vi "CHROMA Set Coupling.vi"(8 "Error In":errorcluster, 10 "Chroma Couple":T1, 11 "CHROMA VISA In":refnum<visa-resource-name>) -> (0 "Error Out":errorcluster, 3 "CHROMA VISA Out":refnum<visa-resource-name>)   [LabVIEW 2020]
uses:
  Type Definition/CHROMA Set Coupling.ctl
  Type Definition/CHROMA Build CMD Type.ctl
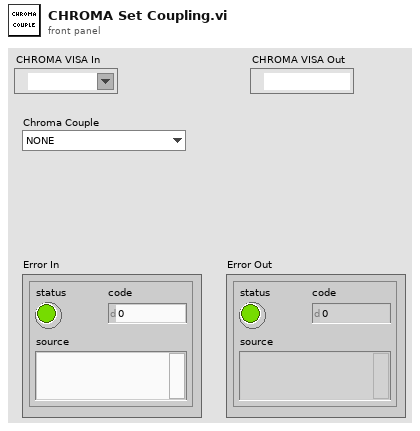
[diagram p1: front panel]
types:
  T1 = typedef "CHROMA Set Coupling.ctl" = enum16{"NONE", "ALL"}
  T2 = typedef "CHROMA Build CMD Type.ctl" = enum16{"Value DBL", "Value I32", "String"}
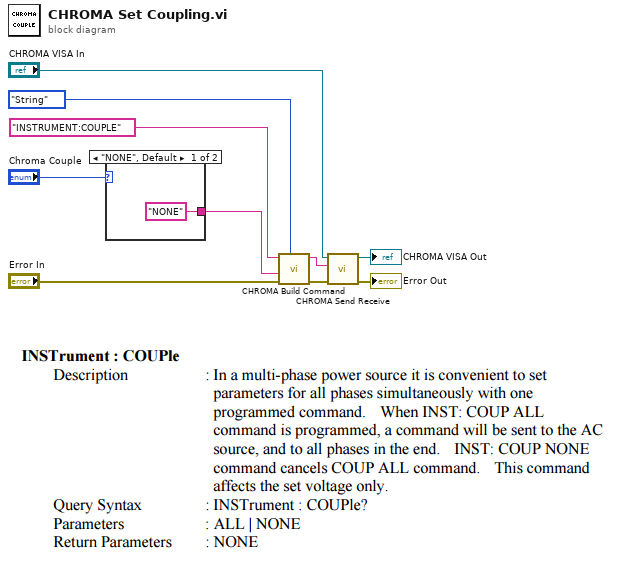
[diagram p0: block diagram]
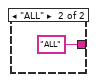
[diagram p2: hidden frame]
diagram:
  n1 = case shown="\"NONE\", Default" "Chroma Couple" {
    tunnel: ["NONE" "ALL"] -> w6
    frame "NONE", Default {
    }
    frame "ALL" {
    }
  }
  n2 = call "CHROMA Build Command.vi"("Build Type"=CHROMA_Build_CMD_Type."String", "Error In"="Error In", "String"=w6, "Partial Command"="INSTRUMENT:COUPLE" ("string to write")) -> ("Error Out"=w9:errorcluster, "Chroma Command"=w5:string)  [unwired: 6 in]
  n3 = call "CHROMA Send Receive.vi"("error in (no error)"=w9, "Send Command"=w5, "CHROMA VISA In"="CHROMA VISA In") -> ("error out"=→"Error Out":errorcluster, "CHROMA VISA Out"=→"CHROMA VISA Out":refnum<visa-resource-name>)  [unwired: 6 in, 1 out]
